vi "2 Parallel Loops Start.vi"() -> ()   [LabVIEW 2015]
uses:
  <vilib>/Analysis/NI_AALBase.lvlib
panel:
  out "Analysis LED":bool
  in  "Stop Button":bool
  out "Histogram":dynamicdata(graph)
  out "STD":dbl(knob) scale=0.0..100.0
  out "Mean":dbl(knob) scale=0.0..100.0
  out "Thermometer":dbl(slide) scale=0.0..100.0
  out "Waveform Chart":dbl(graph)
  in  "Enable Analysis":bool
  in  "Temp":dbl(knob) scale=0.0..100.0
  # "Parallel Loops (Pahse 1)"
  # "Temperature"
  # "Temperature Log"
  # "Statistics"
  # "Statistics"
  # "Analysis \nStatus"
  # "Exit Program"
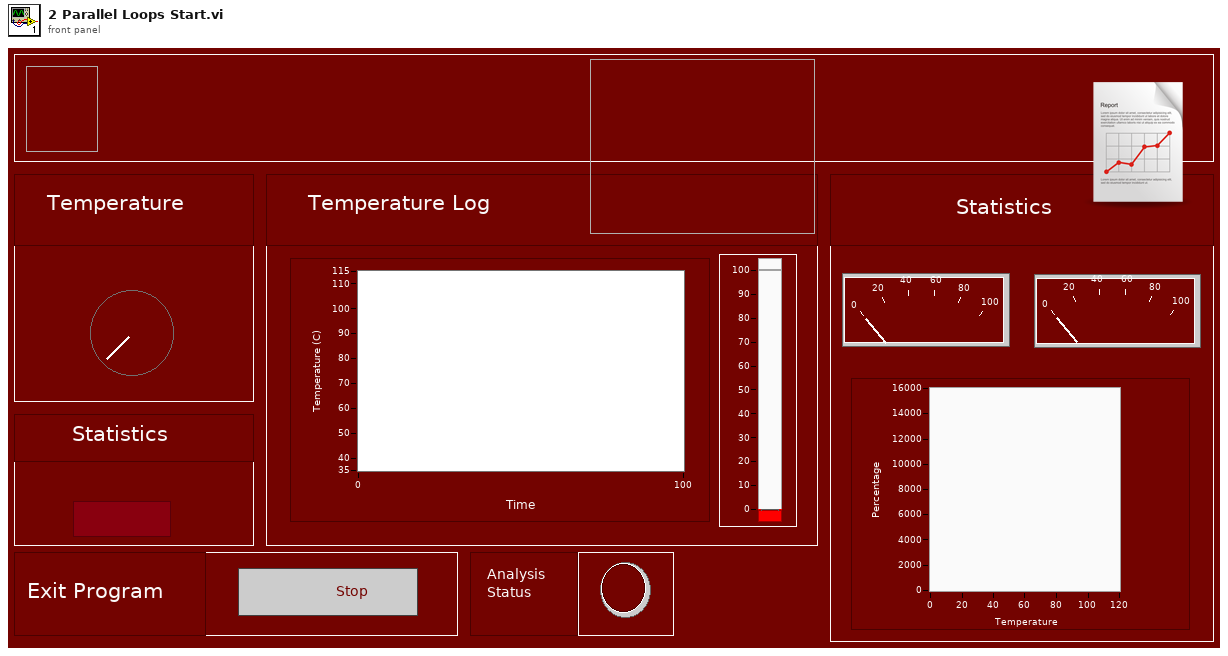
[diagram p1: front panel]
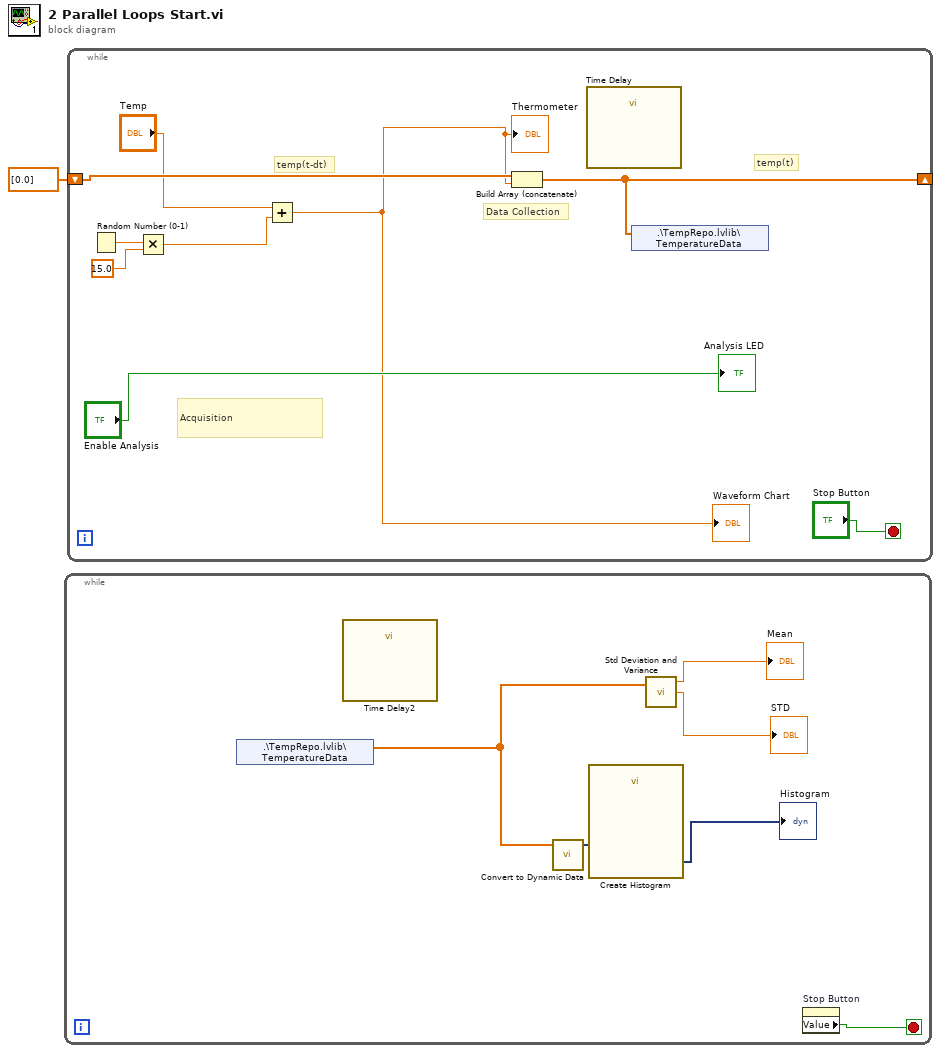
[diagram p0: block diagram]
diagram:
  n1 = while {
    stop <- w7 stop-if-true
    n2 = shared-variable ".\\TempRepo.lvlib\\TemperatureData"() -> (w3:dbl[])  [unwired: 1 in, 1 out]
    n3 = call "Time Delay2"() -> ()  [unwired: 11 in, 1 out]
    n4 = call "Convert to Dynamic Data"("Array"=w3) -> ("Dynamic Data Type"=w2:dynamicdata)  [unwired: 3 in]
    n5 = call "Create Histogram"("Signal"=w2) -> ("Histogram"=→"Histogram":dynamicdata)  [unwired: 9 in, 1 out]
    n6 = call <vilib>:"Std Deviation and Variance.vi"("X"=w3) -> ("mean"=→"Mean":dbl, "standard deviation"=→"STD":dbl)  [unwired: 1 in, 1 out]
    n7 = property on="Stop Button" class="Bool (strict)"() -> ("Value"=w7:bool)  [unwired: 2 in, 2 out]
  }
  n8 = while {
    shift-right: [w8] -> _
    shift-left: dbl[] [0.0] -> [w14]
    stop <- "Stop Button" stop-if-true
    # "Acquisition"
    # "temp(t)"
    # "temp(t-dt)"
    # "Data Collection"
    n9 = Random Number (0-1)() -> (number: 0 to 1=w16:dbl)
    n10 = Multiply(x=w16, y=15.0) -> (x*y=w12:dbl)
    n11 = Add(x="Temp", y=w12) -> (x+y=w9:dbl)
    "Waveform Chart" <- w9
    "Thermometer" <- w9
    n12 = Build Array (concatenate)(w14, w9) -> (w8:dbl[])
    n13 = call "Time Delay"() -> ()  [unwired: 11 in, 1 out]
    n14 = shared-variable ".\\TempRepo.lvlib\\TemperatureData"(w8) -> ()  [unwired: 1 in, 1 out]
    "Analysis LED" <- "Enable Analysis"
  }
